vi "BenchC2_DEV_v111.vi"() -> ()   [LabVIEW 2016]
uses:
  x64/Debug/BERTTA.dll
panel:
  out "element":bool
  out "Started:":string
  in  "SHUTDOWN":bool
  in  "MASTER CONTROL":bool
  in  "Tab Control":T1(tab)
  out "Output File":path caption="selected path"
  in  "Browse folder":path=path "" caption="start path"
  in  "Read Seq":bool
  in  "Save Seq":bool
  in  "Configuration file":path caption="Filename"
  in  "OK Button 2":bool
  out "Boolean":bool
  in  "User (initials)":string
  in  "Project name":string
  in  "Description":string
  out "PUMP1":bool
  out "Target amount":dbl
  out "Scale weight":dbl
  out "Amount now":dbl
  out "Flow rate":dbl
  out "Time to target":dbl format="%<%H:%M:%S>t"
  out "Current step":dbl
  out "Target":dbl
  out "Amount now":dbl
  out "Amount now":dbl
  out "Target":dbl
  out "Current step":dbl
  out "Time to target":dbl format="%<%H:%M:%S>t"
  out "Flow rate":dbl
  out "Amount now":dbl
  out "Scale weight":dbl
  out "Target amount":dbl
  out "PUMP2":bool
  out "Sensor OK 6":bool
  out "Sensor OK 5":bool
  out "Sensor OK 4":bool
  out "Sensor OK 3":bool
  in  "OK Button":bool
  in  "Add comment":string
  out "PUMP3":bool
  out "Target amount":dbl
  out "Scale weight":dbl
  out "Amount now":dbl
  out "Flow rate":dbl
  out "Time to target":dbl format="%<%H:%M:%S>t"
  out "Current step":dbl
  out "Target":dbl
  out "Amount now":dbl
  out "Tr":dbl
  out "Tj in":dbl
  out "Tj out":dbl
  out "T set":dbl
  out "Current step":i32
  out "RPM":dbl
  out "Torque 2":dbl
  out "Waveform Chart 5":dynamicdata(graph)
  out "Waveform Chart 6":dynamicdata(graph)
  out "Waveform Chart 7":dynamicdata(graph)
  out "Table":string[][](table)=[["14.8.2017 18.06.59", "0,000000", "417,670000", "-0,150000", "1,000000", "22,220000", "23,366837", "23,574959", "23,985852", "23,690000", "240,000000", "4,000000", "0,000000", "397,000000", "-397,000000", "1,000000"], ["14.8.2017 18.07.06", "0,000000", "417,640000", "-0,120000", "1,000000", "22,220000", "23,763115", "23,906257", "23,985694", "23,680000", "240,000000", "4,000000", "0,000000", "397,000000", "-397,000000", "1,000000"], ["14.8.2017 18.07.13", "0,000000", "417,640000", "-0,120000", "1,000000", "22,220000", "23,965922", "24,013440", "23,984906", "23,670000", "240,000000", "4,100000", "3,000000", "397,000000", "-397,000000", "1,000000"], ["14.8.2017 18.07.21", "0,000000", "417,640000", "-0,120000", "1,000000", "22,220000", "23,943860", "23,900110", "23,987113", "23,670000", "240,000000", "4,000000", "0,000000", "397,000000", "-397,000000", "1,000000"], ["14.8.2017 18.07.28", "0,000000", "417,640000", "-0,120000", "1,000000", "22,220000", "23,736328", "23,600018", "23,989004", "23,660000", "240,000000", "4,000000", "0,000000", "397,000000", "-397,000000", "1,000000"], ["14.8.2017 18.07.36", "0,000000", "417,640000", "-0,120000", "1,000000", "22,220000", "23,480910", "23,324538", "23,991053", "23,660000", "240,000000", "4,000000", "0,000000", "397,000000", "-397,000000", "1,000000"], ["14.8.2017 18.07.43", "0,000000", "417,640000", "-0,120000", "2,000000", "22,220000", "23,195579", "23,008270", "23,999093", "23,650000", "240,000000", "4,000000", "0,000000", "397,000000", "-397,000000", "1,000000"], ["14.8.2017 18.07.51", "0,000000", "417,650000", "-417,650000", "1,000000", "22,220000", "22,862541", "22,649021", "24,003979", "23,650000", "240,000000", "4,000000", "0,000000", "397,000000", "-397,000000", "2,000000"], ["14.8.2017 18.07.58", "0,000000", "417,640000", "0,010000", "1,000000", "22,220000", "22,541353", "22,354878", "24,005398", "23,650000", "240,000000", "4,000000", "0,000000", "397,000000", "-397,000000", "1,000000"], ["14.8.2017 18.08.06", "0,000000", "417,640000", "0,010000", "1,000000", "22,220000", "22,347931", "22,253738", "24,007605", "23,640000", "240,000000", "4,100000", "0,000000", "397,000000", "-397,000000", "1,000000"], ["14.8.2017 18.08.13", "0,000000", "417,640000", "0,010000", "1,000000", "22,220000", "22,329030", "22,302102", "24,006028", "23,640000", "240,000000", "4,000000", "0,000000", "395,820000", "-395,820000", "1,000000"], ["14.8.2017 18.08.20", "0,000000", "417,640000", "0,010000", "1,000000", "22,220000", "22,466849", "22,511320", "24,002403", "23,630000", "240,000000", "4,000000", "0,000000", "395,830000", "-0,010000", "1,000000"], ["14.8.2017 18.08.28", "0,000000", "417,640000", "0,010000", "1,000000", "22,220000", "22,707062", "22,835101", "24,000984", "23,620000", "240,000000", "4,000000", "0,000000", "395,830000", "-0,010000", "1,000000"], ["14.8.2017 18.08.35", "0,000000", "417,640000", "0,010000", "1,000000", "22,220000", "23,054104", "23,232979", "24,001299", "23,600000", "240,000000", "4,000000", "0,000000", "395,830000", "-0,010000", "1,000000"], ["14.8.2017 18.08.43", "0,000000", "417,640000", "0,010000", "1,000000", "22,220000", "23,412371", "23,522793", "24,002560", "23,590000", "240,000000", "4,000000", "0,000000", "395,820000", "0,000000", "1,000000"], ["14.8.2017 18.08.51", "0,000000", "417,640000", "0,010000", "1,000000", "22,220000", "23,596247", "23,656125", "24,003821", "23,580000", "240,000000", "4,000000", "0,000000", "395,820000", "0,000000", "1,000000"]]
  in  "X scale":i64(slide)=50 scale=0.0..100.0
  in  "Tr/Tj mode selector 2":bool=TRUE
  in  "Tr/Tj mode selector":bool=TRUE
  out "Boolean 4":bool
  out "Boolean 3":bool
  out "Boolean 2":bool
  in  "Reset 6":bool
  in  "Manual/Ramp":bool=TRUE
  in  "Array":dbl[][](array[numeric])=[[20.0, 0.0], [20.0, 0.0], [20.0, 0.0]]
  in  "?":bool
  in  "Time":dbl format="Time to target (min):                %#_g"
  out "Current temp":dbl format="Current temperature (S1):   %#_6g"
  in  "OK Button 3":bool
  out "Sensor OK":bool
  in  "T fail":dbl=20.0 format="Failsafe temperature:              %#_g"
  in  "Setpoint":dbl=20.0 format="Temperature target:                %#_6g"
  out "Waveform Chart":dynamicdata(graph)
  out "T external 2":dbl format="Current temp S2:    %#_g"
  in  "UPDATE TEMP":bool
  in  "Reset 11":bool
  in  "Reset 10":bool
  in  "Tube select":u32(ring) items=["Purple tube", "Yellow tube", " White tube"]
  out "Led11 5":bool
  out "RPM":dbl format="%_4f"
  out "Led5 3":bool
  out "Led4 3":bool
  out "Led3 3":bool
  out "Led2 3":bool
  out "Led1 3":bool
  in  "PumpSeq 4":dbl[][](array[numeric])=[[0.0, 0.0, 0.0, 0.0, 0.0, 0.0, 0.0, 0.0, 0.0, 0.0], [0.0, 0.0, 0.0, 0.0, 0.0, 0.0, 0.0, 0.0, 0.0, 0.0], [0.0, 0.0, 0.0, 0.0, 0.0, 0.0, 0.0, 0.0, 0.0, 0.0], [0.0, 0.0, 0.0, 0.0, 0.0, 0.0, 0.0, 0.0, 0.0, 0.0], [0.0, 0.0, 0.0, 0.0, 0.0, 0.0, 0.0, 0.0, 0.0, 0.0], [0.0, 0.0, 0.0, 0.0, 0.0, 0.0, 0.0, 0.0, 0.0, 0.0], [0.0, 0.0, 0.0, 0.0, 0.0, 0.0, 0.0, 0.0, 0.0, 0.0], [0.0, 0.0, 0.0, 0.0, 0.0, 0.0, 0.0, 0.0, 0.0, 0.0], [0.0, 0.0, 0.0, 0.0, 0.0, 0.0, 0.0, 0.0, 0.0, 0.0], [0.0, 0.0, 0.0, 0.0, 0.0, 0.0, 0.0, 0.0, 0.0, 0.0]]
  in  "?":bool
  out "Flow rate (g/min)":dbl
  out "Scale reading":dbl
  out "Step amount now":dbl
  in  "Grams / min":dbl
  out "Waveform Chart 14":dynamicdata(graph)
  out "Total amount now":dbl
  out "Led11 4":bool
  in  "Reset 5":bool
  out "Elapsed / step":dbl format="%<%H:%M:%S>t"
  out "Time to target":dbl format="%<%H:%M:%S>t"
  in  "OK Button 4":bool
  in  "Grams / min 2":dbl
  in  "?":bool
  out "Led11 7":bool
  out "Led11 6":bool
  in  "PumpSeq 5":dbl[][](array[numeric])=[[0.0, 0.0, 0.0, 0.0, 0.0, 0.0, 0.0, 0.0, 0.0, 0.0], [0.0, 0.0, 0.0, 0.0, 0.0, 0.0, 0.0, 0.0, 0.0, 0.0], [0.0, 0.0, 0.0, 0.0, 0.0, 0.0, 0.0, 0.0, 0.0, 0.0], [0.0, 0.0, 0.0, 0.0, 0.0, 0.0, 0.0, 0.0, 0.0, 0.0], [0.0, 0.0, 0.0, 0.0, 0.0, 0.0, 0.0, 0.0, 0.0, 0.0], [0.0, 0.0, 0.0, 0.0, 0.0, 0.0, 0.0, 0.0, 0.0, 0.0], [0.0, 0.0, 0.0, 0.0, 0.0, 0.0, 0.0, 0.0, 0.0, 0.0], [0.0, 0.0, 0.0, 0.0, 0.0, 0.0, 0.0, 0.0, 0.0, 0.0], [0.0, 0.0, 0.0, 0.0, 0.0, 0.0, 0.0, 0.0, 0.0, 0.0], [0.0, 0.0, 0.0, 0.0, 0.0, 0.0, 0.0, 0.0, 0.0, 0.0]]
  out "Led1 4":bool
  out "Led2 4":bool
  out "Led3 4":bool
  out "Led4 4":bool
  out "Led5 4":bool
  in  "Reset 7":bool
  in  "Tube select 2":u32(ring) items=["Purple tube", "Yellow tube", " White tube"]
  out "Time to target 2":dbl format="%<%H:%M:%S>t"
  out "Elapsed / step 2":dbl format="%<%H:%M:%S>t"
  out "Total amount now 2":dbl
  out "Step amount now 2":dbl
  out "Scale reading 2":dbl
  out "Flow rate (g/min) 2":dbl
  out "RPM 2":dbl format="%_4f"
  in  "Grams / min 3":dbl
  in  "?":bool
  out "Led11 9":bool
  out "Led11 8":bool
  in  "PumpSeq 6":dbl[][](array[numeric])=[[0.0, 0.0, 0.0, 0.0, 0.0, 0.0, 0.0, 0.0, 0.0, 0.0], [0.0, 0.0, 0.0, 0.0, 0.0, 0.0, 0.0, 0.0, 0.0, 0.0], [0.0, 0.0, 0.0, 0.0, 0.0, 0.0, 0.0, 0.0, 0.0, 0.0], [0.0, 0.0, 0.0, 0.0, 0.0, 0.0, 0.0, 0.0, 0.0, 0.0], [0.0, 0.0, 0.0, 0.0, 0.0, 0.0, 0.0, 0.0, 0.0, 0.0], [0.0, 0.0, 0.0, 0.0, 0.0, 0.0, 0.0, 0.0, 0.0, 0.0], [0.0, 0.0, 0.0, 0.0, 0.0, 0.0, 0.0, 0.0, 0.0, 0.0], [0.0, 0.0, 0.0, 0.0, 0.0, 0.0, 0.0, 0.0, 0.0, 0.0], [0.0, 0.0, 0.0, 0.0, 0.0, 0.0, 0.0, 0.0, 0.0, 0.0], [0.0, 0.0, 0.0, 0.0, 0.0, 0.0, 0.0, 0.0, 0.0, 0.0]]
  out "Led1 5":bool
  out "Led2 5":bool
  out "Led3 5":bool
  out "Led4 5":bool
  out "Led5 5":bool
  in  "Reset 8":bool
  in  "Tube select 3":u32(ring) items=["Purple tube", "Yellow tube", " White tube"]
  out "Time to target 3":dbl format="%<%H:%M:%S>t"
  out "Elapsed / step 3":dbl format="%<%H:%M:%S>t"
  out "Total amount now 3":dbl
  out "Step amount now 3":dbl
  out "Scale reading 3":dbl
  out "Flow rate (g/min) 3":dbl
  out "RPM 3":dbl format="%_4f"
  in  "Reset 9":bool
  out "Waveform Chart 16":dynamicdata(graph)
  out "Waveform Chart 17":dynamicdata(graph)
  in  "OK Button 5":bool
  in  "OK Button 6":bool
  in  "?":bool
  in  "Scale port":dbl=5.0
  out "Waveform Chart 15":dynamicdata(graph)
  in  "?":bool
  in  "OK Button 8":bool
  in  "Remote / Manual":bool
  in  "Set RPM":i32
  out "RPM":dbl
  out "Torque":dbl
  out "Waveform Chart 4":dynamicdata(graph)
  in  "OK Button 7":bool
  out "PortDev out":dbl[](array[numeric])
  in  "Save PortDev":bool
  out "PortDev in":dbl[](array[numeric])
  in  "dev1":i32
  in  "dev2":i32
  in  "dev3":i32
  in  "dev4":i32
  in  "dev5":i32
  in  "dev6":i32
  in  "dev8":i32
  in  "port1":i32
  in  "port2":i32
  in  "port3":i32
  in  "port4":i32
  in  "port5":i32
  in  "port6":i32
  in  "port7":i32
  in  "port8":i32
  in  "dev7":i32
  in  "Treshold (T/C)":dbl=0.5
  out "DAQ 9217 (PT100)":errorcluster
  out "Config File":dbl[][](array[numeric])
  in  "Temp Control":tag="cDAQ9188XT-1C3BF2FMod1"
  in  "PAM Control":tag="cDAQ9188XT-1C3BF2FMod7"
  # "Temperature sensor:"
  # "Manual control:"
  # "PUMP & SCALE 1"
  # "STEP"
  # "TOTAL"
  # "PUMP & SCALE 2"
  # "STEP"
  # "TOTAL"
  # "PUMP & SCALE 3"
  # "STEP"
  # "TOTAL"
  # "Temperature control parameter"
  # "Secondary temperature sensor"
  # "Temp target"
  # "Time target"
  # "PAM control"
  # "dev1 and dev2 always to port1 and 2\nport1 = port2 = Lauda\n\ndev3 and dev4 always to port3 and port4\nport3 = port4 = Heidolph"
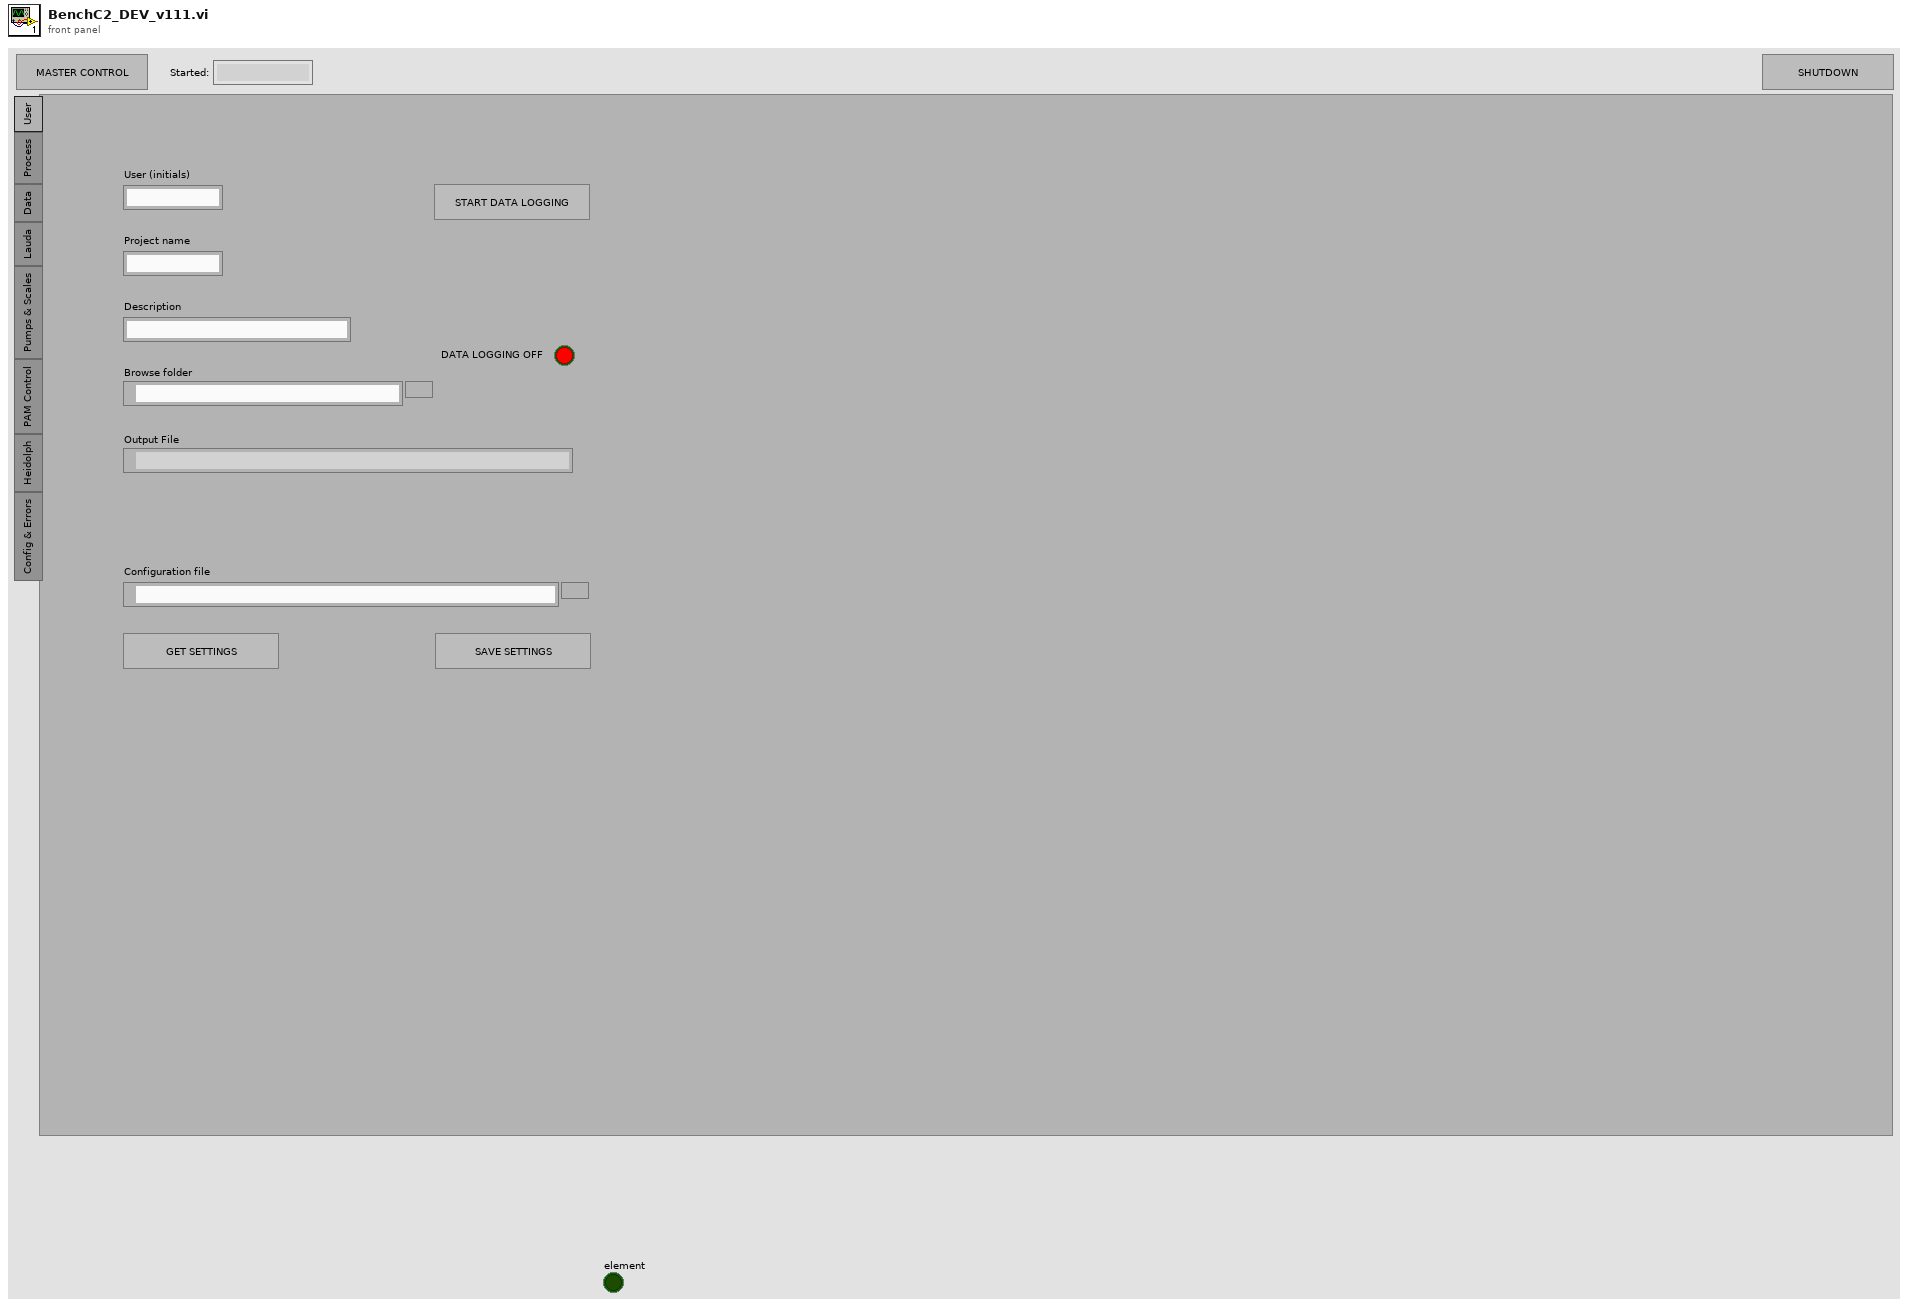
[diagram p1: front panel]
types:
  T1 = enum32{"User", "Process", "Data", "Lauda", "Pumps & Scales", "PAM Control", "Heidolph", "Config & Errors"}
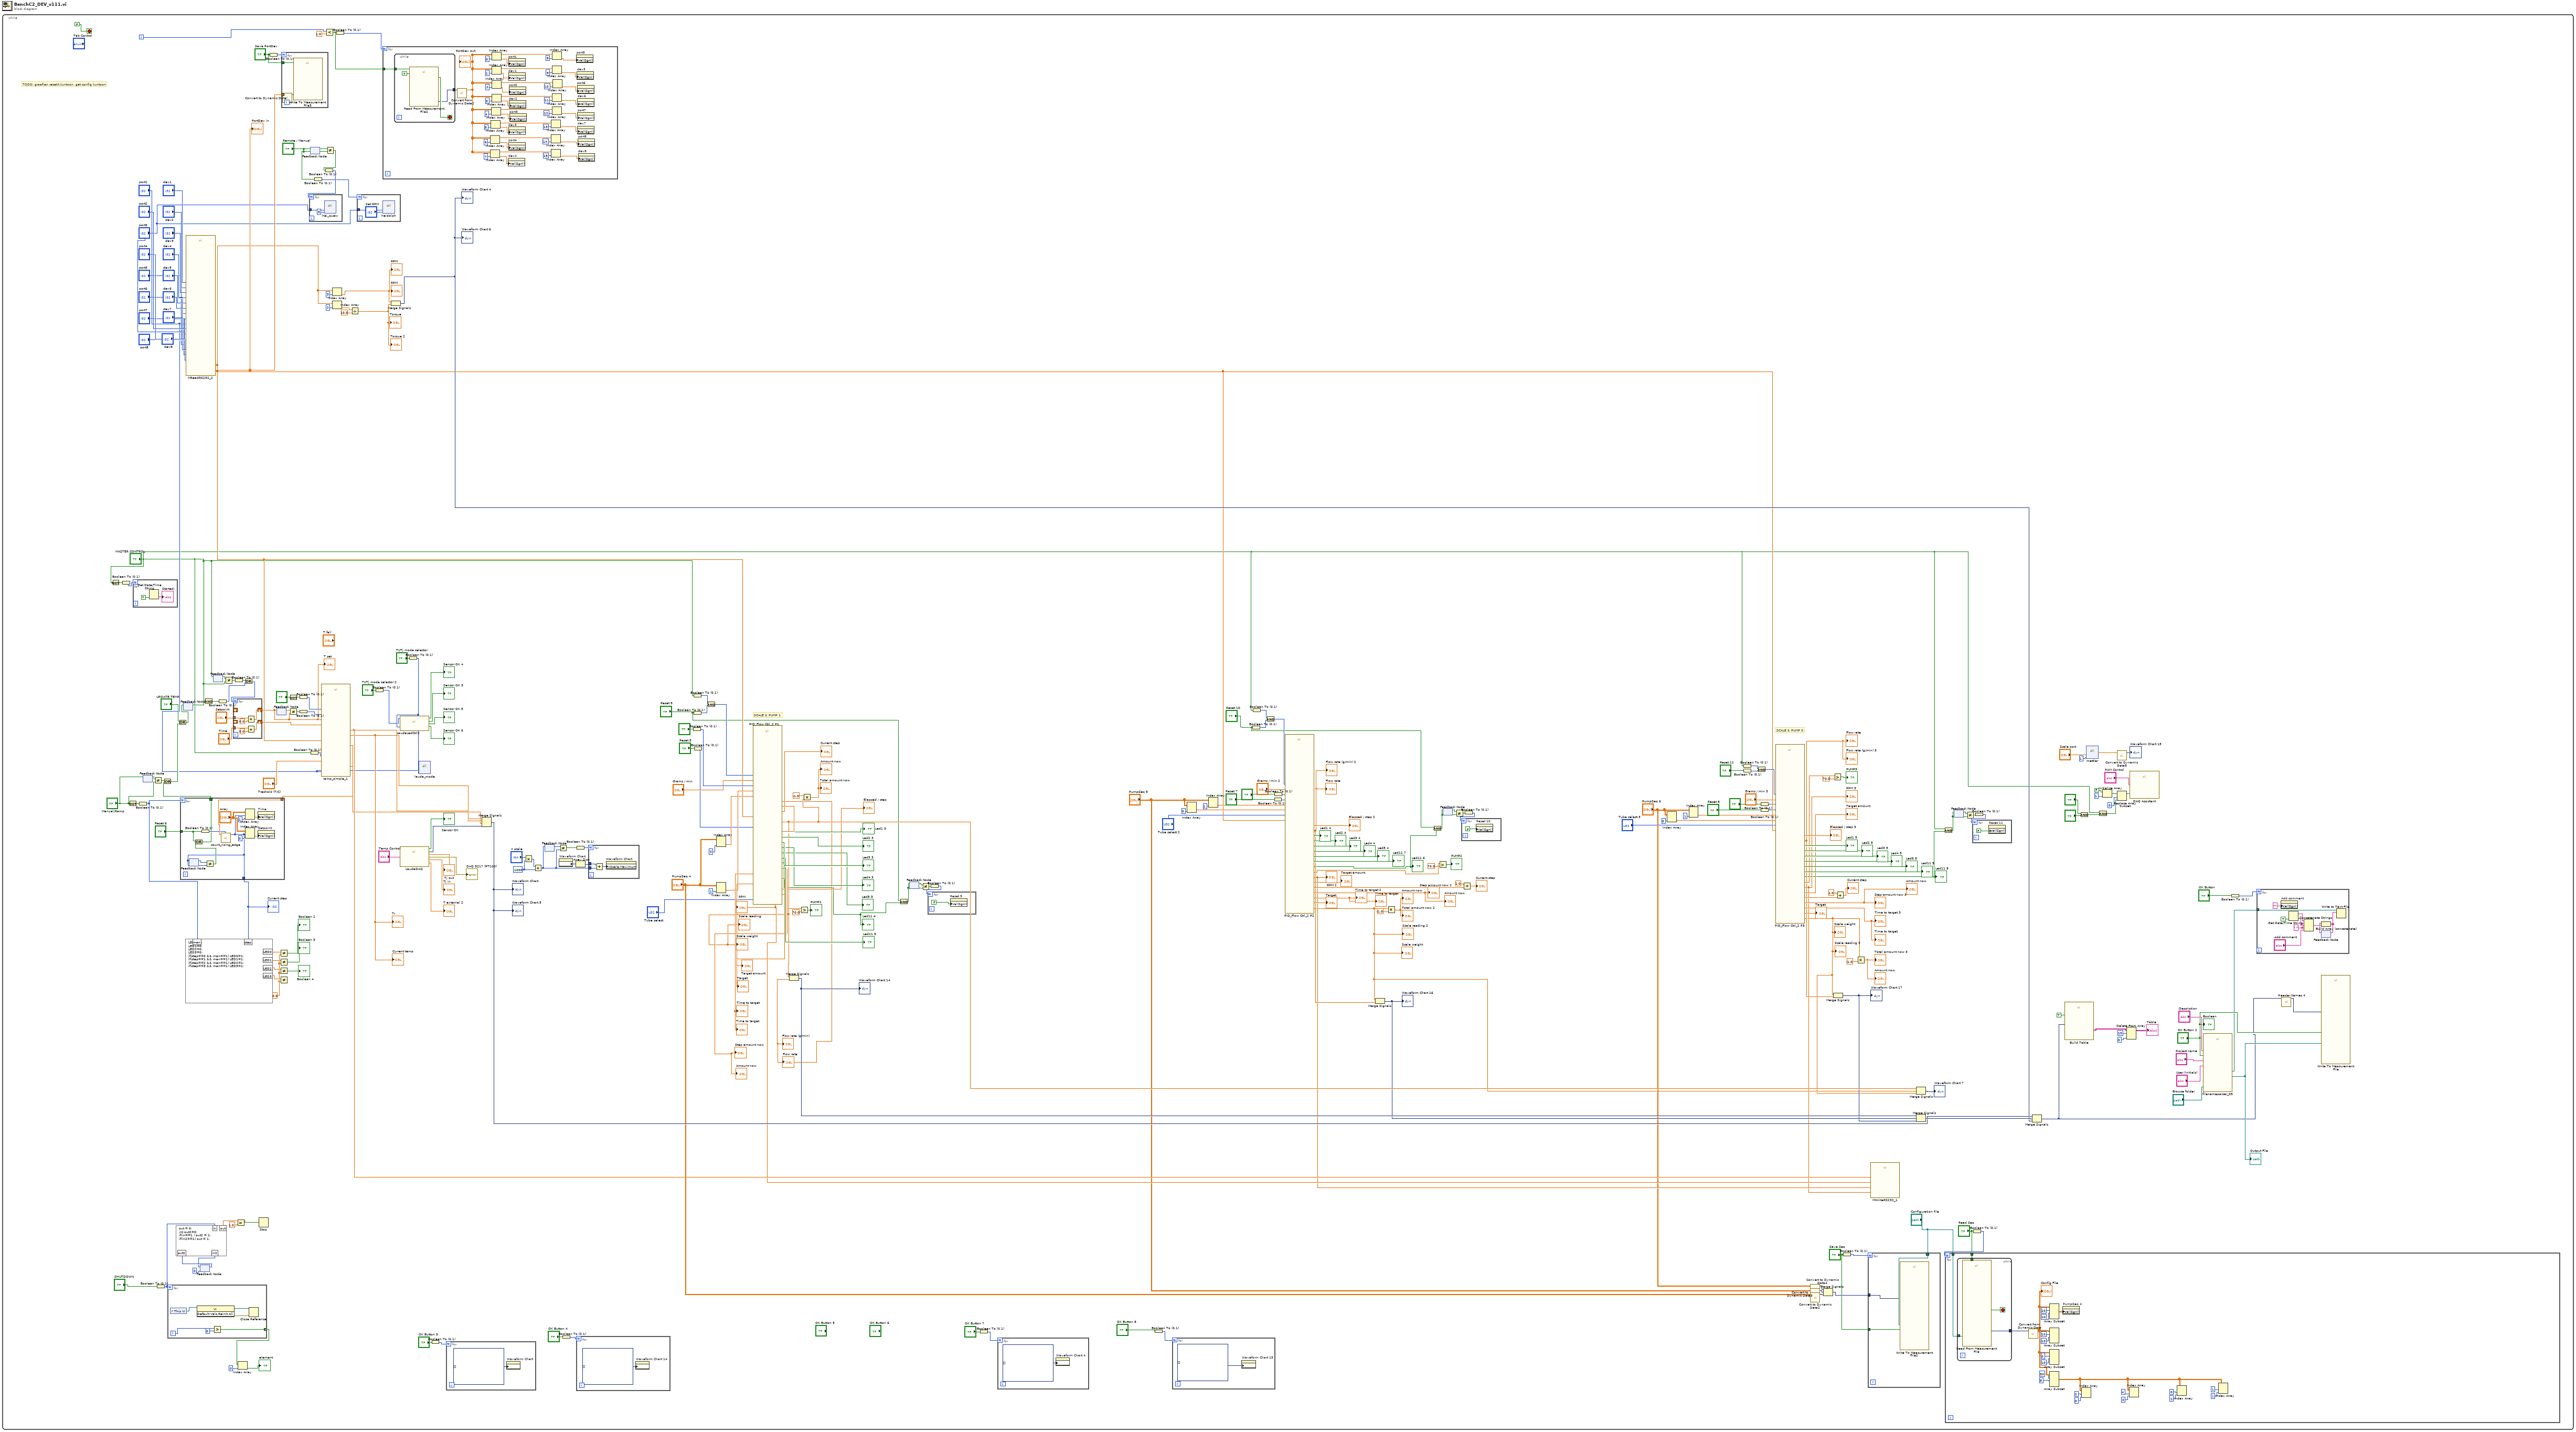
[diagram p0: block diagram]
diagram:
  n1 = while {
    i -> [w188]
    stop <- FALSE stop-if-true
    w121 = i64 1000 ("y")
    w174 = 0.0 ("y")
    # "TODO: graafien resetit kuntoon, get config kuntoon"
    # "SCALE & PUMP 1"
    # "SCALE & PUMP 3"
    n2 = Not(x="MASTER CONTROL") -> (.not. x?=w289:bool)
    n3 = Boolean To (0,1)(Boolean=w289) -> (0, 1=w290:i16)
    n4 = Not(x="Manual/Ramp") -> (.not. x?=w181:bool)
    n5 = for {
      N: w290 -> [_]
      n6 = Get Date/Time String(want seconds? (F)=TRUE) -> (time string=→"Started:":string)  [unwired: 2 in, 1 out]
    }
    n7 = Boolean To (0,1)(Boolean=w181) -> (0, 1=w164:i16)
    n8 = feedback #1() -> (w170:bool)  [unwired: 1 in]
    n9 = feedback-in #1("Manual/Ramp") -> ()
    n10 = Not Equal?(x=w170, y="Manual/Ramp") -> (x != y?=w167:bool)
    n11 = Boolean To (0,1)(Boolean="SHUTDOWN") -> (0, 1=w274:i16)
    n12 = for {
      N: w274 -> [_]
      tunnel: [w408] -> w288 mode=indexing
      i -> [w410]
      n13 = control-ref of="This VI"() -> (w413:refnum<vi>)
      n14 = invoke class="VI" method="Default Vals.Reinit All"(reference=w413) -> (reference out=w411:refnum<vi>, error out=w412:errorcluster)  [unwired: 2 in, 1 out]
      n15 = Greater?(x=w410, y=0) -> (0:w408:bool)
      n16 = Close Reference(reference=w411, error in (no error)=w412) -> ()  [unwired: 1 out]
    }
    n17 = feedback #2() -> (w162:bool)  [unwired: 1 in]
    n18 = call "MReadRS232_2.vi"("port1"="port1", "dev1"="dev1", "port2"="port2", "dev2"="dev2", "port3"="port3", "dev7"="dev7", "dev8"="dev8", "port7"="port7", "port8"="port8", "dev5"="dev5", "port5"="port5", "dev4"="dev4", "dev6"="dev6", "port6"="port6", "port4"="port4", "dev3"="dev3") -> ("output array"=w192:dbl[], "params"=w36:dbl[])  [unwired: 2 in]
    "PortDev in" <- w192
    n19 = feedback #3(0) -> (w272:i32)
    n20 = formula code="out = 0;\nint out2=0;\nif(in==1 ) out2 = 1;\nif(in2==1) out = 1;"("in"=w274, "in2"=w272) -> ("out"=w276:dbl, "out2"=w273:i32)
    n21 = feedback-in #3(w273) -> ()
    n22 = And(x="MASTER CONTROL", y=w162) -> (x .and. y?=w218:bool)
    n23 = feedback #4() -> (w210:bool)  [unwired: 1 in]
    n24 = feedback-in #4("MASTER CONTROL") -> ()
    n25 = Boolean To (0,1)(Boolean=w218) -> (0, 1=w208:i16)
    n26 = Not Equal?(x=w210, y="MASTER CONTROL") -> (x != y?=w209:bool)
    n27 = Boolean To (0,1)(Boolean=w209) -> (0, 1=w207:i16)
    n28 = Equal?(x=w276, y=1.0) -> (x = y?=w275:bool)
    n29 = Index Array(array=w288, index=0) -> (element=→"element":bool)
    n30 = Or(x=w207, y=w208) -> (x .or. y?=w206:i16)
    n31 = for {
      N: w206 -> [_]
      tunnel: "Time" -> [w364]
      shift-right: [w363] -> w219
      shift-left: _ -> [_]
      tunnel: "Setpoint" -> [w361]
      shift-right: [w360] -> w130
      shift-left: _ -> [_]
      n32 = Add(x=w361, y=0.0) -> (x+y=w360:dbl)
      n33 = Add(x=w364, y=0.0) -> (x+y=w363:dbl)
    }
    "T set" <- w130
    n34 = Stop(stop? (T)=w275) -> ()
    n35 = Boolean To (0,1)(Boolean="Save PortDev") -> (0, 1=w191:i16)
    n36 = feedback-in #5(w130) -> ()
    n37 = feedback #5() -> (w217:dbl)  [unwired: 1 in]
    n38 = for {
      N: w191 -> [_]
      tunnel: w192 -> [w359]
      tunnel: "Save PortDev" -> [w357]
      n39 = call "Convert to Dynamic Data"("Array"=w359) -> ("Dynamic Data Type"=w358:dynamicdata)  [unwired: 3 in]
      n40 = call "Write To Measurement File3"("Signals"=w358, "Reset"=w357) -> ()  [unwired: 15 in, 3 out]
    }
    n41 = Not(x="?") -> (.not. x?=w213:bool)
    n42 = Not Equal?(x=w217, y=w130) -> (x != y?=w216:bool)
    n43 = Boolean To (0,1)(Boolean=w213) -> (0, 1=w215:i16)
    n44 = Boolean To (0,1)(Boolean=w216) -> (0, 1=w211:i16)
    n45 = Boolean To (0,1)(Boolean="MASTER CONTROL") -> (0, 1=w212:i16)
    n46 = feedback-in #6("Remote / Manual") -> ()
    n47 = feedback #6() -> (w159:bool)  [unwired: 1 in]
    n48 = Boolean To (0,1)(Boolean="Remote / Manual") -> (0, 1=w157:i16)
    n49 = call "ramp_simple_1.vi"("pause"=w215, "time_set"=w219, "array"=w36, "reset"=w211, "master"=w212, "T_sp"=w130, "treshold"="Treshold (T/C)", "port"="port1") -> ("Tin"=w222:dbl, "Tr"=w223:dbl, "target_reached"=w179:dbl, "T control"=w224:dbl)  [unwired: 3 in, 1 out]
    "Tr" <- w223
    "Current temp" <- w223
    n50 = for {
      N: w164 -> [_]
      tunnel: w179 -> [w316]
      tunnel: [w306] -> w168
      tunnel: "Reset 6" -> [w308]
      tunnel: [w309] -> w131
      n51 = feedback #7() -> (w310:i32)  [unwired: 1 in]
      n52 = Boolean To (0,1)(Boolean=w308) -> (0, 1=w311:i16)
      n53 = call "count_rising_edge.vi"("reset"=w311, "target_reached"=w316) -> ("element 2"=w309:i32)  [unwired: 9 in]
      n54 = feedback-in #7(w309) -> ()
      n55 = Not Equal?(x=w310, y=w309) -> (x != y?=w307:bool)
      n56 = Or(x=w308, y=w307) -> (x .or. y?=w306:bool)
      n57 = Index Array(array="Array", index (row)=w309, index (col)=1 ("disabled index (col)")) -> (element=w312:dbl)
      n58 = Index Array(array="Array", index (row)=w309, index (col)=0 ("disabled index (col)")) -> (element=w313:dbl)
      n59 = property on="Time" class="DigNum (strict)"("Val(Sgnl)"=w312) -> ()  [unwired: 2 in, 2 out]
      n60 = property on="Setpoint" class="DigNum (strict)"("Val(Sgnl)"=w313) -> ()  [unwired: 2 in, 2 out]
    }
    "Current step" <- w131
    n61 = Or(x=w167, y=w168) -> (x .or. y?=w166:bool)
    n62 = Or(x="UPDATE TEMP", y=w166) -> (x .or. y?=w163:bool)
    n63 = feedback-in #2(w163) -> ()
    n64 = formula code="LED0=0;\nLED1=0;\nLED2=0;\nLED3=0;\nif(step==0 && man==1) LED0=1;\nif(step==1 && man==1) LED1=1;\nif(step==2 && man==1) LED2=1;\nif(step==3 && man==1) LED3=1;"("step"=w131, "man"=w164) -> ("LED0"=w178:dbl, "LED1"=w177:dbl, "LED2"=w176:dbl, "LED3"=w175:dbl)
    n65 = Not Equal?(x=w178, y=w174) -> (x != y?=→"Boolean 2":bool)
    n66 = Not Equal?(x=w177, y=w174) -> (x != y?=→"Boolean 3":bool)
    n67 = Not Equal?(x=w176, y=w174) -> (x != y?=→"Boolean 4":bool)
    n68 = Not Equal?(x=w175, y=w174) -> ()  [unwired: 1 out]
    n69 = Less?(x=w188, y=1.0) -> (x < y?=w186:bool)
    n70 = Not Equal?(x=w159, y="Remote / Manual") -> (x != y?=w158:bool)
    n71 = Boolean To (0,1)(Boolean=w158) -> (0, 1=w160:i16)
    n72 = for {
      N: w160 -> [_]
      tunnel: "port3" -> [w304]
      n73 = dll-call lib="C:/Users/shresplab/OneDrive - Kemira Oyj/Documents/GitHub/Bertta/BERTTA/x64/Debug/BERTTA.dll" fn="hei_query"("port"=w304, "q"=5) -> ()  [unwired: 6 in, 2 out]
    }
    n74 = Index Array(array=w36, index=3) -> (element=w152:dbl)
    "RPM" <- w152
    "RPM" <- w152
    n75 = Index Array(array=w36, index=2) -> (element=w154:dbl)
    n76 = Boolean To (0,1)(Boolean=w186) -> (0, 1=w187:i16)
    n77 = Divide(x=w154, y=10.0) -> (x/y=w151:dbl)
    "Torque" <- w151
    "Torque 2" <- w151
    n78 = for {
      N: w157 -> [_]
      tunnel: "port3" -> [w302]
      n79 = dll-call lib="C:/Users/shresplab/OneDrive - Kemira Oyj/Documents/GitHub/Bertta/BERTTA/x64/Debug/BERTTA.dll" fn="heidolph"("port"=w302, "speed"="Set RPM") -> ()  [unwired: 6 in, 2 out]
    }
    n80 = Boolean To (0,1)(Boolean="Tr/Tj mode selector 2") -> (0, 1=w125:i16)
    n81 = for {
      N: w187 -> [_]
      tunnel: w186 -> [w352]
      n82 = while {
        tunnel: [w355] -> w351
        tunnel: w352 -> [w353]
        stop <- w356 stop-if-true
        n83 = call "Read From Measurement File2"("Enable"=TRUE, "Reset"=w353) -> ("Signals"=w355:dynamicdata, "EOF?"=w356:bool)  [unwired: 4 in, 4 out]
      }
      n84 = call "Convert from Dynamic Data2"("Dynamic Data Type"=w351) -> ("Array"=w334:dbl[])  [unwired: 3 in]
      "PortDev out" <- w334
      n85 = Index Array(array=w334, index=6) -> (element=w327:dbl)
      n86 = Index Array(array=w334, index=7) -> (element=w326:dbl)
      n87 = Index Array(array=w334, index=5) -> (element=w328:dbl)
      n88 = Index Array(array=w334, index=4) -> (element=w329:dbl)
      n89 = Index Array(array=w334, index=0) -> (element=w333:dbl)
      n90 = Index Array(array=w334, index=1) -> (element=w332:dbl)
      n91 = Index Array(array=w334, index=3) -> (element=w330:dbl)
      n92 = Index Array(array=w334, index=2) -> (element=w331:dbl)
      n93 = property on="dev4" class="DigNum (strict)"("Val(Sgnl)"=w326) -> ()  [unwired: 2 in, 2 out]
      n94 = property on="dev3" class="DigNum (strict)"("Val(Sgnl)"=w328) -> ()  [unwired: 2 in, 2 out]
      n95 = property on="port4" class="DigNum (strict)"("Val(Sgnl)"=w327) -> ()  [unwired: 2 in, 2 out]
      n96 = property on="port1" class="DigNum (strict)"("Val(Sgnl)"=w333) -> ()  [unwired: 2 in, 2 out]
      n97 = property on="dev1" class="DigNum (strict)"("Val(Sgnl)"=w332) -> ()  [unwired: 2 in, 2 out]
      n98 = property on="port2" class="DigNum (strict)"("Val(Sgnl)"=w331) -> ()  [unwired: 2 in, 2 out]
      n99 = property on="dev2" class="DigNum (strict)"("Val(Sgnl)"=w330) -> ()  [unwired: 2 in, 2 out]
      n100 = property on="port3" class="DigNum (strict)"("Val(Sgnl)"=w329) -> ()  [unwired: 2 in, 2 out]
      n101 = Index Array(array=w334, index=14) -> (element=w319:dbl)
      n102 = Index Array(array=w334, index=15) -> (element=w318:dbl)
      n103 = Index Array(array=w334, index=13) -> (element=w320:dbl)
      n104 = Index Array(array=w334, index=12) -> (element=w321:dbl)
      n105 = Index Array(array=w334, index=8) -> (element=w325:dbl)
      n106 = Index Array(array=w334, index=9) -> (element=w324:dbl)
      n107 = Index Array(array=w334, index=11) -> (element=w322:dbl)
      n108 = Index Array(array=w334, index=10) -> (element=w323:dbl)
      n109 = property on="port5" class="DigNum (strict)"("Val(Sgnl)"=w325) -> ()  [unwired: 2 in, 2 out]
      n110 = property on="dev5" class="DigNum (strict)"("Val(Sgnl)"=w324) -> ()  [unwired: 2 in, 2 out]
      n111 = property on="port6" class="DigNum (strict)"("Val(Sgnl)"=w323) -> ()  [unwired: 2 in, 2 out]
      n112 = property on="dev6" class="DigNum (strict)"("Val(Sgnl)"=w322) -> ()  [unwired: 2 in, 2 out]
      n113 = property on="port7" class="DigNum (strict)"("Val(Sgnl)"=w321) -> ()  [unwired: 2 in, 2 out]
      n114 = property on="dev7" class="DigNum (strict)"("Val(Sgnl)"=w320) -> ()  [unwired: 2 in, 2 out]
      n115 = property on="port8" class="DigNum (strict)"("Val(Sgnl)"=w319) -> ()  [unwired: 2 in, 2 out]
      n116 = property on="dev8" class="DigNum (strict)"("Val(Sgnl)"=w318) -> ()  [unwired: 2 in, 2 out]
    }
    n117 = Merge Signals(w152, w151) -> (w150:dynamicdata)
    "Waveform Chart 4" <- w150
    "Waveform Chart 6" <- w150
    n118 = call "LaudaDAQ.vi"("device name"="Temp Control") -> ("error out"=→"DAQ 9217 (PT100)":errorcluster, 1:"Tj out"=→"Tj out":dbl, "data"=w258:dynamicdata, "Sensor OK"=→"Sensor OK":bool, 4:"Tj out"=→"Tj in":dbl, "T external 2"=→"T external 2":dbl)  [unwired: 5 in]
    n119 = Boolean To (0,1)(Boolean="Tr/Tj mode selector") -> (0, 1=w127:i16)
    n120 = call "LaudaLedCtrl2.vi"("ctrl_mode"=w127, "T ext / T ext in"=w125) -> ("Sensor OK 5"=→"Sensor OK 5":bool, "Sensor OK 3"=→"Sensor OK 3":bool, "Sensor OK 4"=→"Sensor OK 4":bool, "Sensor OK 6"=→"Sensor OK 6":bool)  [unwired: 6 in]
    n121 = dll-call lib="C:/Users/shresplab/OneDrive - Kemira Oyj/Documents/GitHub/Bertta/BERTTA/x64/Debug/BERTTA.dll" fn="lauda_mode"("port"="port1", "mode"=w127) -> ()  [unwired: 6 in, 2 out]
    n122 = Boolean To (0,1)(Boolean="OK Button 3") -> (0, 1=w231:i16)
    n123 = for {
      N: w231 -> [_]
      n124 = property on="Waveform Chart" class="WFChart (strict)"("History Data"=dynamicdata[] []) -> ()  [unwired: 2 in, 2 out]
    }
    n125 = Merge Signals(w224, w223, w222, w258) -> (w259:dynamicdata)
    "Waveform Chart" <- w259
    "Waveform Chart 5" <- w259
    n126 = Multiply(x="X scale", y=w121) -> (x*y=w122:i64)
    n127 = Add(x=w122, y=w121) -> (x+y=w117:i64)
    n128 = feedback-in #8(w117) -> ()
    n129 = feedback #8() -> (w120:i64)  [unwired: 1 in]
    n130 = Not Equal?(x=w120, y=w117) -> (x != y?=w119:bool)
    n131 = property on="Waveform Chart" class="WFChart (strict)"() -> ("History Data"=w124:dynamicdata[])  [unwired: 2 in, 2 out]
    n132 = Boolean To (0,1)(Boolean="OK Button 4") -> (0, 1=w229:i16)
    n133 = Boolean To (0,1)(Boolean=w119) -> (0, 1=w116:i16)
    n134 = Array Size(array=w124) -> (size(s)=w118:i32)
    n135 = for {
      N: w229 -> [_]
      n136 = property on="Waveform Chart 14" class="WFChart (strict)"("History Data"=dynamicdata[] []) -> ()  [unwired: 2 in, 2 out]
    }
    n137 = for {
      N: w116 -> [_]
      tunnel: w118 -> [w300]
      tunnel: w117 -> [w299]
      n138 = Add(x=w300, y=w299) -> (x+y=w298:i64)
      n139 = property on="Waveform Chart" class="WFChart (strict)"("XScale.Maximum"=w298) -> ()  [unwired: 2 in, 2 out]
    }
    n140 = Boolean To (0,1)(Boolean="?") -> (0, 1=w115:i16)
    n141 = Boolean To (0,1)(Boolean="Reset 9") -> (0, 1=w87:i16)
    n142 = Boolean To (0,1)(Boolean="MASTER CONTROL") -> (0, 1=w113:i16)
    n143 = Boolean To (0,1)(Boolean="Reset 5") -> (0, 1=w108:i16)
    n144 = And(x=w113, y=w87) -> (x .and. y?=w112:i16)
    n145 = Index Array(array="PumpSeq 4", index (col)=0) -> (element=w110:dbl[])  [unwired: 1 in]
    n146 = Index Array(array="PumpSeq 4", index (col)=1) -> (element=w111:dbl[])  [unwired: 1 in]
    n147 = call "PID_Flow Ctrl_2 P1.vi"("weight"=w36, "Setpoint_W"=w110, "Setpoint_T"=w111, "FrManual"="Grams / min", "enable"=w112, "manual"=w115, "reset"=w108, "tube"="Tube select") -> ("elapsed_step"=→"Elapsed / step":dbl, "total_target"=→"Target":dbl, "Setpoint_W"=→"Target amount":dbl, "LED_stop"=w86:bool, "RPM"=w109:dbl, "LED1"=→"Led1 3":bool, "LED4"=→"Led4 3":bool, "LED2"=→"Led2 3":bool, "step_amount"=→"Amount now" →"Step amount now":dbl, "LED3"=→"Led3 3":bool, "LED5"=→"Led5 3":bool, "weight"=w97:dbl, "time_to_target"=→"Time to target" →"Time to target":dbl, "PumpCTRL"=w91:dbl, "step"=→"Current step":dbl, "LED_manual"=→"Led11 5":bool, "FR"=w88:dbl)  [unwired: 3 in]
    "Flow rate" <- w88
    "Scale weight" <- w97
    "Led11 4" <- w86
    "Scale reading" <- w97
    "Flow rate (g/min)" <- w88
    "RPM" <- w109
    n148 = Merge Signals(w97, w88) -> (w261:dynamicdata)
    "Waveform Chart 14" <- w261
    n149 = Greater?(x=w91, y=70.0) -> (0:→"PUMP1":bool)
    n150 = Multiply(x=-1.0, y=w97) -> (x*y=→"Amount now" →"Total amount now":dbl)
    n151 = And(x="Reset 9", y=w86) -> (x .and. y?=w84:bool)
    n152 = feedback #9() -> (w85:bool)  [unwired: 1 in]
    n153 = feedback-in #9(w84) -> ()
    n154 = Not Equal?(x=w85, y=w84) -> (x != y?=w83:bool)
    n155 = Boolean To (0,1)(Boolean=w83) -> (0, 1=w82:i16)
    n156 = for {
      N: w82 -> [_]
      n157 = property on="Reset 9" class="Bool (strict)"("Val(Sgnl)"=FALSE ("Value (Signaling)")) -> ()  [unwired: 2 in, 2 out]
    }
    n158 = Boolean To (0,1)(Boolean="OK Button 7") -> (0, 1=w227:i16)
    n159 = for {
      N: w227 -> [_]
      n160 = property on="Waveform Chart 4" class="WFChart (strict)"("History Data"=dynamicdata[] []) -> ()  [unwired: 2 in, 2 out]
    }
    n161 = Boolean To (0,1)(Boolean="OK Button 8") -> (0, 1=w147:i16)
    n162 = for {
      N: w147 -> [_]
      n163 = property on="Waveform Chart 15" class="WFChart (strict)"("History Data"=dynamicdata[] []) -> ()  [unwired: 2 in, 2 out]
    }
    n164 = Index Array(array="PumpSeq 5", index (col)=0) -> (element=w64:dbl[])  [unwired: 1 in]
    n165 = Index Array(array="PumpSeq 5", index (col)=1) -> (element=w65:dbl[])  [unwired: 1 in]
    n166 = Boolean To (0,1)(Boolean="Reset 10") -> (0, 1=w80:i16)
    n167 = Boolean To (0,1)(Boolean="MASTER CONTROL") -> (0, 1=w81:i16)
    n168 = And(x=w81, y=w80) -> (x .and. y?=w79:i16)
    n169 = Boolean To (0,1)(Boolean="Reset 7") -> (0, 1=w69:i16)
    n170 = Boolean To (0,1)(Boolean="?") -> (0, 1=w71:i16)
    n171 = call "PID_Flow Ctrl_2 P2.vi"("weight"=w36, "Setpoint_W"=w64, "Setpoint_T"=w65, "FrManual"="Grams / min 2", "enable"=w79, "manual"=w71, "reset"=w69, "tube"="Tube select 2") -> ("elapsed_step"=→"Elapsed / step 2":dbl, "total_target"=→"Target":dbl, "Setpoint_W"=→"Target amount":dbl, "LED_stop"=w46:bool, "RPM"=w51:dbl, "LED1"=→"Led1 4":bool, "LED4"=→"Led4 4":bool, "LED2"=→"Led2 4":bool, "step_amount"=→"Amount now" →"Step amount now 2":dbl, "LED3"=→"Led3 4":bool, "LED5"=→"Led5 4":bool, "weight"=w12:dbl, "time_to_target"=→"Time to target" →"Time to target 2":dbl, "PumpCTRL"=w54:dbl, "step"=w59:dbl, "LED_manual"=→"Led11 7":bool, "FR"=w52:dbl)  [unwired: 3 in]
    "Scale weight" <- w12
    "Flow rate" <- w52
    "Led11 6" <- w46
    "Scale reading 2" <- w12
    "Flow rate (g/min) 2" <- w52
    "RPM 2" <- w51
    n172 = Merge Signals(w12, w52) -> (w53:dynamicdata)
    "Waveform Chart 16" <- w53
    n173 = Multiply(x=w12, y=-1.0) -> (x*y=→"Amount now" →"Total amount now 2":dbl)
    n174 = And(x="Reset 10", y=w46) -> (x .and. y?=w49:bool)
    n175 = Greater?(x=w54, y=70.0) -> (0:→"PUMP2":bool)
    n176 = feedback #10() -> (w50:bool)  [unwired: 1 in]
    n177 = feedback-in #10(w49) -> ()
    n178 = Not Equal?(x=w50, y=w49) -> (x != y?=w48:bool)
    n179 = Add(x=1.0, y=w59) -> (x+y=→"Current step":dbl)
    n180 = Boolean To (0,1)(Boolean=w48) -> (0, 1=w47:i16)
    n181 = for {
      N: w47 -> [_]
      n182 = property on="Reset 10" class="Bool (strict)"("Val(Sgnl)"=FALSE ("Value (Signaling)")) -> ()  [unwired: 2 in, 2 out]
    }
    n183 = Index Array(array="PumpSeq 6", index (col)=0) -> (element=w30:dbl[])  [unwired: 1 in]
    n184 = Index Array(array="PumpSeq 6", index (col)=1) -> (element=w31:dbl[])  [unwired: 1 in]
    n185 = Boolean To (0,1)(Boolean="MASTER CONTROL") -> (0, 1=w39:i16)
    n186 = Boolean To (0,1)(Boolean="Reset 11") -> (0, 1=w38:i16)
    n187 = And(x=w39, y=w38) -> (x .and. y?=w37:i16)
    n188 = Boolean To (0,1)(Boolean="?") -> (0, 1=w29:i16)
    n189 = Boolean To (0,1)(Boolean="Reset 8") -> (0, 1=w27:i16)
    n190 = call "PID_Flow Ctrl_2 P3.vi"("weight"=w36, "Setpoint_W"=w30, "Setpoint_T"=w31, "FrManual"="Grams / min 3", "enable"=w37, "manual"=w29, "reset"=w27, "tube"="Tube select 3") -> ("elapsed_step"=→"Elapsed / step 3":dbl, "total_target"=→"Target":dbl, "Setpoint_W"=→"Target amount":dbl, "LED_stop"=w5:bool, "RPM"=w10:dbl, "LED1"=→"Led1 5":bool, "LED4"=→"Led4 5":bool, "LED2"=→"Led2 5":bool, "step_amount"=→"Amount now" →"Step amount now 3":dbl, "LED3"=→"Led3 5":bool, "LED5"=→"Led5 5":bool, "weight"=w11:dbl, "time_to_target"=→"Time to target" →"Time to target 3":dbl, "PumpCTRL"=w24:dbl, "step"=w22:dbl, "LED_manual"=→"Led11 9":bool, "FR"=w16:dbl)  [unwired: 3 in]
    "Scale weight" <- w11
    "Flow rate" <- w16
    "Led11 8" <- w5
    "Scale reading 3" <- w11
    "Flow rate (g/min) 3" <- w16
    "RPM 3" <- w10
    n191 = call "Convert to Dynamic Data4"("2D Array"="PumpSeq 6") -> ("Dynamic Data Type"=w237:dynamicdata)  [unwired: 3 in]
    n192 = call "Convert to Dynamic Data3"("2D Array"="PumpSeq 5") -> ("Dynamic Data Type"=w238:dynamicdata)  [unwired: 3 in]
    n193 = call "Convert to Dynamic Data2"("2D Array"="PumpSeq 4") -> ("Dynamic Data Type"=w240:dynamicdata)  [unwired: 3 in]
    n194 = Merge Signals(w237, w238, w240) -> (w239:dynamicdata)
    n195 = Greater?(x=w24, y=70.0) -> (0:→"PUMP3":bool)
    n196 = Merge Signals(w11, w16) -> (w15:dynamicdata)
    "Waveform Chart 17" <- w15
    n197 = Add(x=1.0, y=w22) -> (x+y=→"Current step":dbl)
    n198 = Boolean To (0,1)(Boolean="Save Seq") -> (0, 1=w236:i16)
    n199 = Multiply(x=w11, y=-1.0) -> (x*y=→"Amount now" →"Total amount now 3":dbl)
    n200 = for {
      N: w236 -> [_]
      tunnel: w239 -> [w406]
      tunnel: "Configuration file" -> [w407]
      tunnel: "Save Seq" -> [w405]
      n201 = call "Write To Measurement File2"("Signals"=w406, "Reset"=w405, "Filename"=w407) -> ()  [unwired: 14 in, 3 out]
    }
    n202 = call "MWriteRS232_1.vi"("P3"=w10, "P2"=w51, "P1"=w109, "LAUDA"=w224) -> ()  [unwired: 8 in]
    n203 = Merge Signals(w261, w53, w15) -> (w260:dynamicdata)
    n204 = Merge Signals(w97, w12, w11) -> (→"Waveform Chart 7":dynamicdata)
    n205 = And(x="MASTER CONTROL", y=w5) -> (x .and. y?=w8:bool)
    n206 = feedback #11() -> (w9:bool)  [unwired: 1 in]
    n207 = feedback-in #11(w8) -> ()
    n208 = Not Equal?(x=w9, y=w8) -> (x != y?=w7:bool)
    n209 = Boolean To (0,1)(Boolean="Read Seq") -> (0, 1=w235:i16)
    n210 = for {
      N: w235 -> [_]
      tunnel: "Configuration file" -> [w380]
      tunnel: "Read Seq" -> [w379]
      n211 = while {
        tunnel: [w404] -> w400
        tunnel: w380 -> [w403]
        tunnel: w379 -> [w401]
        stop <- w402 stop-if-true
        n212 = call "Read From Measurement File"("Filename"=w403, "Reset"=w401) -> ("Signals"=w404:dynamicdata, "EOF?"=w402:bool)  [unwired: 4 in, 4 out]
      }
      n213 = call "Convert from Dynamic Data"("Dynamic Data Type"=w400) -> ("Array"=w392:dbl[][])  [unwired: 3 in]
      "Config File" <- w392
      n214 = Array Subset(array=w392, index (row)=20 ("index"), length (row)=10 ("length")) -> (w397:dbl[][])  [unwired: 2 in]
      n215 = Array Subset(array=w392, index (row)=10 ("index"), length (row)=10 ("length")) -> ()  [unwired: 2 in, 1 out]
      n216 = Array Subset(array=w392, index (row)=0 ("index"), length (row)=10 ("length")) -> ()  [unwired: 2 in, 1 out]
      n217 = Array Subset(array=w392, index (row)=30 ("index"), length (row)=8 ("length")) -> (w381:dbl[][])  [unwired: 2 in]
      n218 = property on="PumpSeq 4" class="Arr (strict)"("Val(Sgnl)"=w397) -> ()  [unwired: 2 in, 2 out]
      n219 = Index Array(array=w381, index (row)=2, index (col)=0 ("disabled index (col)")) -> ()  [unwired: 1 out]
      n220 = Index Array(array=w381, index (row)=4, index (col)=0 ("disabled index (col)")) -> ()  [unwired: 1 out]
      n221 = Index Array(array=w381, index (row)=0, index (col)=1 ("disabled index (col)")) -> ()  [unwired: 1 out]
      n222 = Index Array(array=w381, index (row)=1, index (col)=1 ("disabled index (col)")) -> ()  [unwired: 1 out]
    }
    n223 = Boolean To (0,1)(Boolean=w7) -> (0, 1=w6:i16)
    n224 = for {
      N: w6 -> [_]
      n225 = property on="Reset 11" class="Bool (strict)"("Val(Sgnl)"=FALSE ("Value (Signaling)")) -> ()  [unwired: 2 in, 2 out]
    }
    n226 = Merge Signals(w259, w260, w150) -> (w184:dynamicdata)
    n227 = call "Build Table"("Include time data"=TRUE, "Signals"=w184) -> ("Table"=w284:string[][])  [unwired: 3 in, 6 out]
    n228 = And(x="?", y="?") -> (x .and. y?=w139:bool)
    n229 = dll-call lib="C:/Users/shresplab/OneDrive - Kemira Oyj/Documents/GitHub/Bertta/BERTTA/x64/Debug/BERTTA.dll" fn="mettler"("port"="Scale port", "msg"=1) -> ("return type"=w133:dbl)  [unwired: 5 in, 2 out]
    n230 = And(x="MASTER CONTROL", y=w139) -> (x .and. y?=w136:bool)
    n231 = Initialize Array(FALSE, 1 ("dimension size")) -> (w138:bool[])
    n232 = Replace Array Subset(array=w138, new element=w136, index=0) -> (w135:bool[])
    n233 = call "Convert to Dynamic Data5"("Double"=w133) -> ("Dynamic Data Type"=→"Waveform Chart 15":dynamicdata)  [unwired: 3 in]
    n234 = Delete From Array(array=w284, length=13, index (col)=0 ("index (row)")) -> (array with subset deleted=→"Table":string[][])  [unwired: 1 in, 1 out]
    n235 = call "DAQ Assistant"("data"=w135, "device name"="PAM Control") -> ()  [unwired: 16 in, 2 out]
    n236 = call "filenameparser_09.vi"("Description"="Description", "start path"="Browse folder", "Project name"="Project name", "User (initials)"="User (initials)", "OK Button in"="OK Button 2") -> ("appended path 2"=w225:path, "appended path"=w280:path)  [unwired: 4 in, 1 out]
    "Output File" <- w225
    n237 = Boolean To (0,1)(Boolean="OK Button") -> (0, 1=w279:i16)
    n238 = for {
      N: w279 -> [_]
      tunnel: w280 -> [w371]
      w375 = " " ("string")
      n239 = property on="Add comment" class="Str"("Val(Sgnl)"="" ("Value (Signaling)")) -> ()  [unwired: 2 in, 2 out]
      n240 = Get Date/Time String(want seconds? (F)=TRUE) -> (date string=w378:string, time string=w376:string)  [unwired: 2 in]
      n241 = Concatenate Strings(w378, w375, w376, w375, "Add comment") -> (w374:string)
      n242 = feedback #12() -> (w373:string[])  [unwired: 1 in]
      n243 = Build Array (concatenate)(w373, w374) -> (w372:string[])
      n244 = feedback-in #12(w372) -> ()
      n245 = Write to Text File(file (use dialog)=w371, text=w372) -> ()  [unwired: 2 in, 3 out]
    }
    n246 = call "Header Names 4.vi"("Dynamic Data"=w184) -> ("Signals Out"=w185:dynamicdata)  [unwired: 10 in]
    n247 = call "Write To Measurement File"("Signals"=w185, "Enable"="OK Button 2", "Filename"=w225) -> ()  [unwired: 14 in, 3 out]
    "Boolean" <- "OK Button 2"
  }
